vi "20220106_Counter - Continuous Output.vi"() -> ()   [LabVIEW 2021]
doc: "This example demonstrates how to continuously generate digital pulses using a counter output."
uses:
  <vilib>/Utility/error.llb/DialogType.ctl
  <vilib>/DAQmx/create/channels.llb/DAQmx Create Channel (CO-Pulse Generation-Frequency).vi
  <vilib>/DAQmx/configure/timing.llb/DAQmx Timing (Implicit).vi
  <resource>/objmgr/daqmx.rc
panel:
  in  "DO4":tag="Dev1/ctr0"
  out "Actual Duty Cycle 4":dbl
  out "Actual Frequency 4":dbl
  in  "Duty Cycle4":dbl=0.5 format="%.6f"
  in  "Frequency4":dbl=1.0 format="%.6f"
  in  "Output Terminal4":tag="/Dev1/PFI12"
  out "Actual Duty Cycle":dbl
  out "Actual Frequency":dbl
  in  "Duty Cycle1":dbl=0.5 format="%.6f"
  in  "Frequency1":dbl=1.0 format="%.6f"
  in  "Output Terminal1":tag="/Dev1/PFI12"
  in  "Stop":bool
  in  "DO1":tag="Dev1/ctr0"
  # "Channel Settings"
  # "Channel Settings"
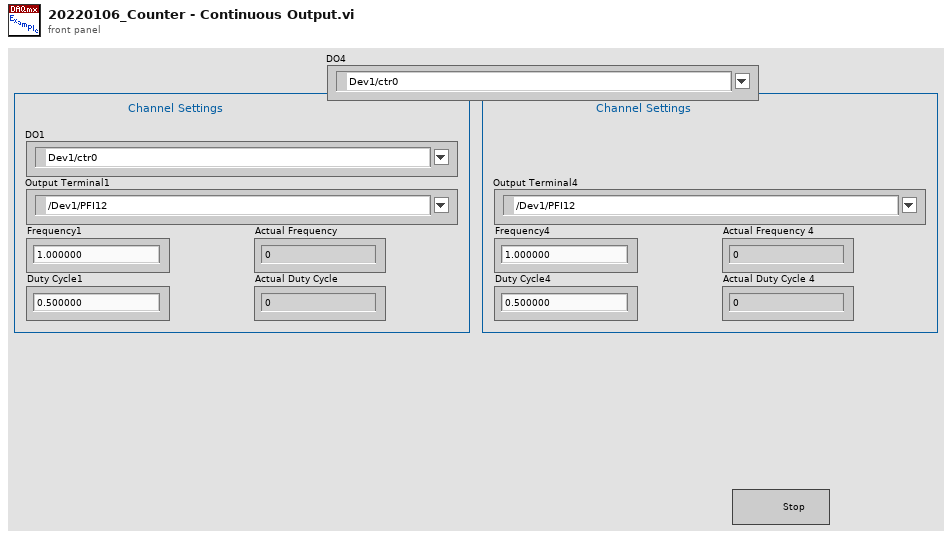
[diagram p1: front panel]
types:
  T1 = typedef "DialogType.ctl" = u16
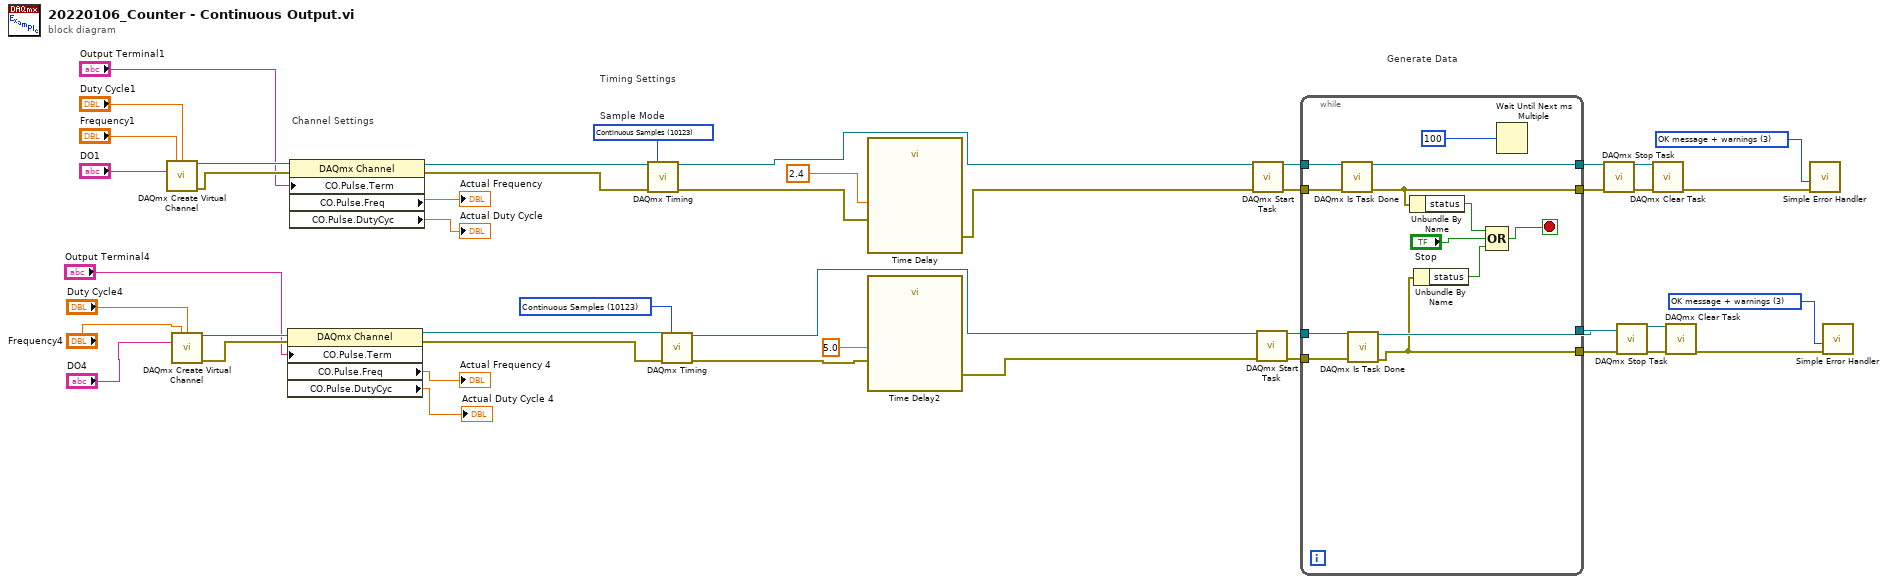
[diagram p0: block diagram]
diagram:
  w7 = T1 3 items=["no dialog", "OK message", "continue or stop message", "OK message + warnings", "continue/stop + warnings"] ("type of dialog (OK msg:1)")
  w14 = 10123 items=["Finite Samples"=10178, "Continuous Samples"=10123, "Hardware Timed Single Point"=12522] ("sample mode")
  w28 = T1 3 items=["no dialog", "OK message", "continue or stop message", "OK message + warnings", "continue/stop + warnings"] ("type of dialog (OK msg:1)")
  w46 = 10123 items=["Finite Samples"=10178, "Continuous Samples"=10123, "Hardware Timed Single Point"=12522]  # Sample Mode
  # "Generate Data"
  # "Timing Settings"
  # "Channel Settings"
  n1 = call-poly <vilib>:"DAQmx Create Virtual Channel.vi"("frequency"="Frequency1", "duty cycle"="Duty Cycle1", "counter"="DO1") -> ("task out"=w41:refnum<k21>, "error out"=w40:errorcluster)  [unwired: 11 in]
  n2 = call-poly <vilib>:"DAQmx Create Virtual Channel.vi"("frequency"="Frequency4", "duty cycle"="Duty Cycle4", "counter"="DO4") -> ("task out"=w21:refnum<k21>, "error out"=w20:errorcluster)  [unwired: 11 in]
  n3 = property class="DAQmx Channel"(reference=w21, error in=w20, "CO.Pulse.Term"="Output Terminal4") -> (reference out=w16:refnum<k21>, error out=w15:errorcluster, "CO.Pulse.Freq"=→"Actual Frequency 4":dbl, "CO.Pulse.DutyCyc"=→"Actual Duty Cycle 4":dbl)
  n4 = property class="DAQmx Channel"(reference=w41, error in=w40, "CO.Pulse.Term"="Output Terminal1") -> (reference out=w37:refnum<k21>, error out=w38:errorcluster, "CO.Pulse.Freq"=→"Actual Frequency":dbl, "CO.Pulse.DutyCyc"=→"Actual Duty Cycle":dbl)
  n5 = call-poly <vilib>:"DAQmx Timing.vi"("task/channels in"=w37, "sample mode"=w46, "error in"=w38) -> ("task out"=w26:refnum<k21>, "error out"=w25:errorcluster)  [unwired: 11 in]
  n6 = call-poly <vilib>:"DAQmx Timing.vi"("task/channels in"=w16, "sample mode"=w14, "error in"=w15) -> ("task out"=w10:refnum<k21>, "error out"=w12:errorcluster)  [unwired: 11 in]
  n7 = call "Time Delay"("error in (no error)"=w25, "Delay Time (s)"=2.4) -> ("error out"=w24:errorcluster)  [unwired: 9 in]
  n8 = call "Time Delay2"("error in (no error)"=w12, "Delay Time (s)"=5.0) -> ("error out"=w11:errorcluster)  [unwired: 9 in]
  n9 = call <vilib>:"DAQmx Start Task.vi"("task/channels in"=w26, "error in"=w24) -> ("task out"=w45:refnum<k21>, "error out"=w44:errorcluster)  [unwired: 12 in]
  n10 = call <vilib>:"DAQmx Start Task.vi"("task/channels in"=w10, "error in"=w11) -> ("task out"=w9:refnum<k21>, "error out"=w8:errorcluster)  [unwired: 12 in]
  n11 = while {
    tunnel: w45 -> [w59]
    tunnel: w44 -> [w58]
    tunnel: [w56] -> w29
    tunnel: [w57] -> w30
    tunnel: w9 -> [w54]
    tunnel: w8 -> [w53]
    tunnel: [w52] -> w3
    tunnel: [w49] -> w2
    stop <- w47 stop-if-true
    n12 = call <vilib>:"DAQmx Is Task Done.vi"("task/channels in"=w59, "error in"=w58) -> ("task out"=w57:refnum<k21>, "error out"=w56:errorcluster)  [unwired: 11 in, 1 out]
    n13 = call <vilib>:"DAQmx Is Task Done.vi"("task/channels in"=w54, "error in"=w53) -> ("task out"=w52:refnum<k21>, "error out"=w49:errorcluster)  [unwired: 11 in, 1 out]
    n14 = Unbundle By Name(w56) -> ("status"=w51:bool)
    n15 = Unbundle By Name(w49) -> ("status"=w48:bool)
    n16 = Compound Arithmetic op=OR(w51, "Stop", w48) -> (w47:bool)
    n17 = Wait Until Next ms Multiple(millisecond multiple=u32 100) -> ()  [unwired: 1 out]
  }
  n18 = call <vilib>:"DAQmx Stop Task.vi"("task/channels in"=w30, "error in"=w29) -> ("task out"=w32:refnum<k21>, "error out"=w31:errorcluster)  [unwired: 12 in]
  n19 = call <vilib>:"DAQmx Stop Task.vi"("task/channels in"=w3, "error in"=w2) -> ("task out"=w5:refnum<k21>, "error out"=w6:errorcluster)  [unwired: 12 in]
  n20 = call <vilib>:"DAQmx Clear Task.vi"("task in"=w32, "error in"=w31) -> ("error out"=w43:errorcluster)  [unwired: 13 in]
  n21 = call <vilib>:"DAQmx Clear Task.vi"("task in"=w5, "error in"=w6) -> ("error out"=w4:errorcluster)  [unwired: 13 in]
  n22 = call <vilib>:"Simple Error Handler.vi"("type of dialog (OK msg:1)"=w28, "error in (no error)"=w43) -> ()  [unwired: 3 in, 5 out]
  n23 = call <vilib>:"Simple Error Handler.vi"("type of dialog (OK msg:1)"=w7, "error in (no error)"=w4) -> ()  [unwired: 3 in, 5 out]
